vi "File Exists__ogtk.vi"   [LabVIEW 2019]
doc: "Checks to see whether a path exists on disk and whether it is a directory."
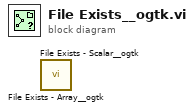
[diagram p0: block diagram]
diagram:
  n1 = call "File Exists - Array__ogtk.vi"() -> ()  [unwired: 7 in, 2 out]
  n2 = call "File Exists - Scalar__ogtk.vi"() -> ()  [unwired: 7 in, 2 out]
